vi "ni579x FPGA Align 2.vi"(0 "sync.resources":T1, 1 "sync.meas.Reference Clock":refnum<k21>) -> (4 "sync.resources":T1)   [LabVIEW 2015, in "ni579x Synchronization v1 FPGA.lvlib"]
doc: "Align the targets participating in synchronization. This must occur before a signal can be synchronized.\n\nThere are two flavors of alignment to chose from -- Host Align and FPGA Align. The two flavors produce the same quality of synchronization, but differ in requirements and versatility of operation.\n\nWhen using <B>ni579x FPGA Align 2</B>, the Single Cycle Timed Loop (SCTL) rate (that this VI is in) must be an integer multiple of the <B>sync.cptr.Reference Clock</B> rate, and the SCTL clock must have a fixed phase relationship to the reference clock. Each target performs its alignment independently, so FPGA Align does not require an FPGA I/O line. It's also possible to use FPGA Align without host interaction. FPGA Align has 100% repeatability if-and-only-if the target-to-target phase relationship is low and does not change.\n\nWhen using <B>ni579x Host Align 2</B>, the SCTL rate may be arbitrary (yet still must have a fixed phase relationship to the other targets). The CPTR period may also be arbitrary. This alignment process is coordinated by the host, and requires an FPGA I/O line for orchestration. Host Align has 100% repeatability; if the hardware configuration remains constant, so will the level of synchronization.\n\n<B>Input Parameters</B>\n\n<B>sync.resources</B> identifies the Synchronization instance. 'sync.resources' is obtained from the ni579x Create VI of this library.\n\n<B>sync.meas.Reference Clock</B> is used by the measurement logic as the \"start\" signal.\n\nWhen using 'ni579x FPGA Align', the 'sync.meas.Reference Clock' must be the same clock that the target's FPGA Clock is locked to. This is commonly PXI_Clk10.\n\n<B>Output Parameters</B>\n\n<B>sync.resources</B> is the same instance that was passed in for 'sync.resources'."
uses:
  <instrlib>/ni579x/Synchronization/v1/FPGA/ni579x Synchronization v1 FPGA.lvlib
  <vilib>/eio/EIONode/EIONode.xnode
  <instrlib>/_niInstr/Basic Elements/v1/FPGA/niInstr Basic Elements v1 FPGA.lvlib
  <instrlib>/_niInstr/TDC/v1/FPGA/niInstr Overclocked TDC v1 FPGA.lvlib
  <vilib>/rvi/eio/common/nirviEmuTemplateMethod_errors.vi
  <instrlib>/ni579x/Synchronization/v1/FPGA/Implementation/Resources.ctl
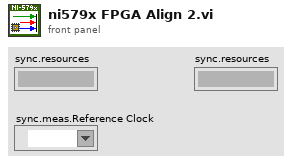
[diagram p1: front panel]
types:
  T1 = typedef "ni579x Synchronization v1 FPGA.lvlib/Resources.ctl" = cluster{"master":refnum<k21>, "meas.enable":refnum<k21>, "meas.ready":refnum<k21>, "meas.arm":refnum<k21>, "meas.valid":refnum<k21>, "meas.value":refnum<k21>, "meas.oversample clock":refnum<k21>, "meas.oversample factor":refnum<k21>, "cptr":refnum<k21>, "cptr.adjust":refnum<k21>, "cptr.period":refnum<k21>}
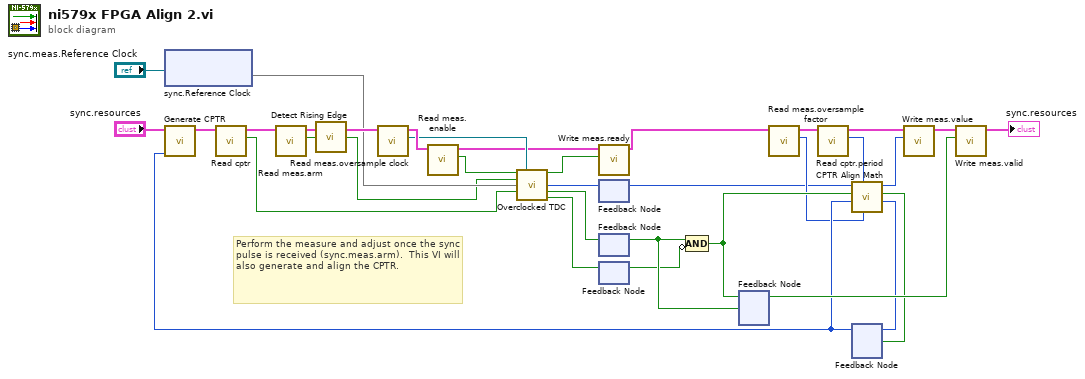
[diagram p0: block diagram]
diagram:
  # "Perform the measure and adjust once the sync pulse is received (sync.meas.arm).  This VI will also generate and align the CPTR."
  n1 = xnode ("sync.Reference Clock")("FPGA I/O In"="sync.meas.Reference Clock") -> ("I/O Item"=w11)  [unwired: 1 out]
  n2 = feedback #1() -> (w7:u16)  [unwired: 1 in]
  n3 = feedback #2() -> (w3:bool)  [unwired: 1 in]
  n4 = feedback #3() -> (w1:bool)  [unwired: 1 in]
  n5 = Compound Arithmetic op=AND(w3, invert w1) -> (w24:bool)
  n6 = feedback #4() -> (w33:bool)  [unwired: 1 in]
  n7 = feedback-in #4(w24, w3) -> ()
  n8 = feedback #5() -> (w28:u16)  [unwired: 1 in]
  n9 = call <instrlib>:"Generate CPTR.vi"("sync.cptr.adjust"=w28, "sync.resources"="sync.resources") -> ("sync.resources"=w29:T1)  [unwired: 9 in]
  n10 = call <instrlib>:"Read cptr.vi"("sync.resources"=w29) -> ("cptr"=w9:bool, "sync.resources"=w30:T1)  [unwired: 9 in]
  n11 = call <instrlib>:"Read meas.arm.vi"("sync.resources"=w30) -> ("meas.arm"=w31:bool, "sync.resources"=w19:T1)  [unwired: 9 in]
  n12 = call <instrlib>:"Detect Rising Edge.vi"("signal"=w31) -> ("edge detected"=w10:bool)  [unwired: 14 in]
  n13 = call <instrlib>:"Read meas.oversample clock.vi"("sync.resources"=w19) -> ("meas.oversample clock"=w12:refnum<k21>, "sync.resources"=w15:T1)  [unwired: 9 in]
  n14 = call <instrlib>:"Read meas.enable.vi"("sync.resources"=w15) -> ("meas.enable"=w14:bool, "sync.resources"=w6:T1)  [unwired: 9 in]
  n15 = call <instrlib>:"Overclocked TDC.vi"("enable"=w14, "counter clock"=w12, "arm"=w10, "start"=w11, "stop"=w9) -> ("ready"=w13:bool, "count"=w8:u16, "count valid"=w4:bool, "rollover"=w2:bool)  [unwired: 6 in, 1 out]
  n16 = call <instrlib>:"Write meas.ready.vi"("meas.ready"=w13, "sync.resources"=w6) -> ("sync.resources"=w5:T1)  [unwired: 9 in]
  n17 = feedback-in #1(w8) -> ()
  n18 = feedback-in #2(w4) -> ()
  n19 = feedback-in #3(w2) -> ()
  n20 = call <instrlib>:"Read meas.oversample factor.vi"("sync.resources"=w5) -> ("meas.oversample factor"=w16:u16, "sync.resources"=w17:T1)  [unwired: 9 in]
  n21 = call <instrlib>:"Read cptr.period.vi"("sync.resources"=w17) -> ("cptr.period"=w22:u16, "sync.resources"=w23:T1)  [unwired: 9 in]
  n22 = call <instrlib>:"CPTR Align Math.vi"("sync.meas.oversample factor"=w16, "sync.cptr.period"=w22, "sync.cptr.adjust"=w28, "measurement valid"=w24, "measurement"=w7) -> ("new sync.cptr.adjust"=w27:u16, "new sync.cptr.adjust valid"=w18:bool, "measurement (in sample clocks)"=w25:u16)  [unwired: 4 in]
  n23 = feedback-in #5(w27, w18) -> ()
  n24 = call <instrlib>:"Write meas.value.vi"("meas.value"=w25, "sync.resources"=w23) -> ("sync.resources"=w26:T1)  [unwired: 9 in]
  n25 = call <instrlib>:"Write meas.valid.vi"("meas.valid"=w33, "sync.resources"=w26) -> ("sync.resources"=→"sync.resources":T1)  [unwired: 9 in]
